vi "runTCP.vi"(8 "error in (no error)":errorcluster, 11 "MonoCommunicator in":refnum<class "MonoCommunicator.lvclass">) -> (0 "error out":errorcluster, 3 "MonoCommunicator out":refnum<class "MonoCommunicator.lvclass">)   [LabVIEW 2016, in "MonoCommunicator.lvclass"]
uses:
  MonoCommunicator.lvclass
  MonoCommunicator.lvclass/MonoCommunicator.ctl
  ts_labview_tcp/TCPServer/TCPServer.lvclass
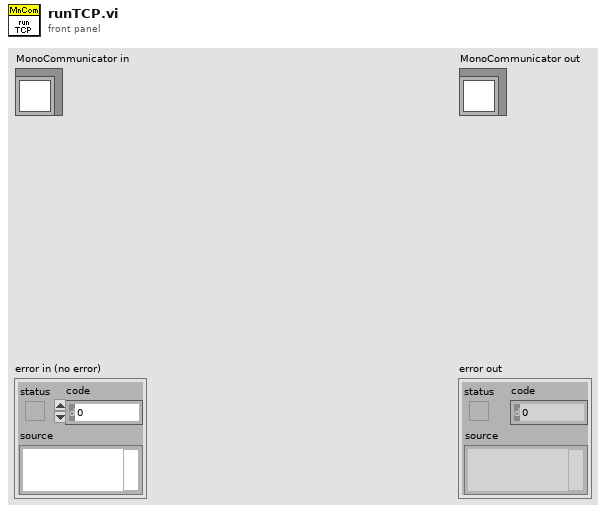
[diagram p1: front panel]
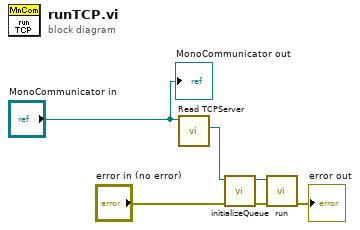
[diagram p0: block diagram]
diagram:
  n1 = call "Read TCPServer.vi"("MonoCommunicator in"="MonoCommunicator in") -> ("TCPServer.lvclass"=w2:refnum<class "TCPServer.lvclass">)  [unwired: 8 in, 2 out]
  n2 = call-dynamic "initializeQueue.vi"("error in (no error)"="error in (no error)", "TCPCommunicator in"=w2) -> ("error out"=w6:errorcluster, "TCPCommunicator out"=w3:refnum<class "TCPServer.lvclass">)  [unwired: 8 in]
  n3 = call-dynamic "run.vi"("error in (no error)"=w6, "TCPServer in"=w3) -> ("error out"=→"error out":errorcluster)  [unwired: 8 in, 1 out]
  "MonoCommunicator out" <- "MonoCommunicator in"
